vi "zadanie_4.vi"() -> ()   [LabVIEW 2020]
panel:
  in  "stop":bool
  out "S.O.S.":bool
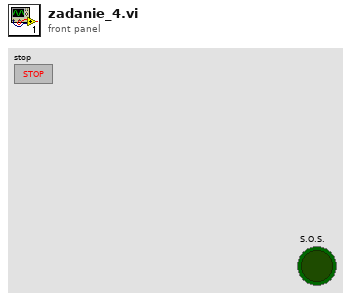
[diagram p1: front panel]
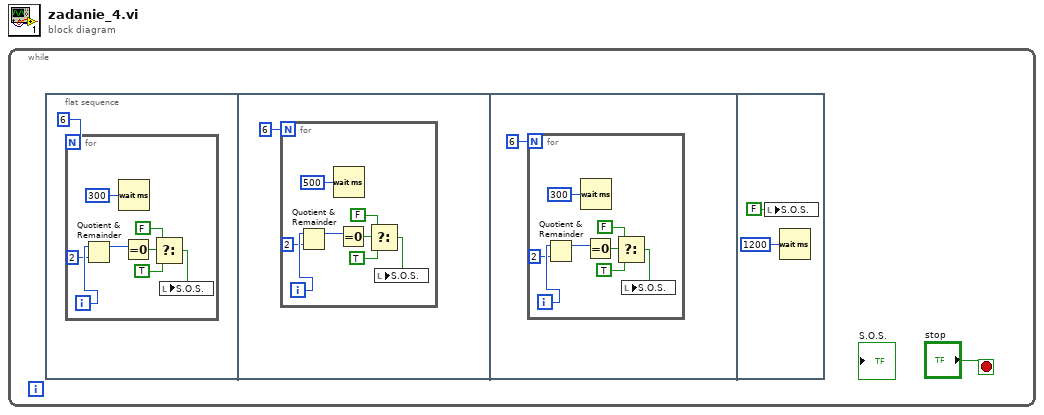
[diagram p0: block diagram]
diagram:
  n1 = while {
    stop <- "stop" stop-if-true
    n2 = flat-sequence {
      frame #0 {
        n3 = for {
          N: 6 -> [_]
          i -> [w9]
          n4 = Quotient & Remainder(x=w9, y=2) -> (x-y*floor(x/y)=w7:i32)  [unwired: 1 out]
          n5 = Wait (ms)(milliseconds to wait=u32 300) -> ()  [unwired: 1 out]
          n6 = Equal To 0?(x=w7) -> (x = 0?=w6:bool)
          n7 = Select(t=FALSE, s=w6, f=TRUE) -> (s? t:f=w5:bool)
          n8 = local write "S.O.S."(w5) -> ()
        }
      }
      frame #1 {
        n9 = for {
          N: 6 -> [_]
          i -> [w18]
          n10 = Quotient & Remainder(x=w18, y=2) -> (x-y*floor(x/y)=w16:i32)  [unwired: 1 out]
          n11 = Wait (ms)(milliseconds to wait=u32 500) -> ()  [unwired: 1 out]
          n12 = Equal To 0?(x=w16) -> (x = 0?=w15:bool)
          n13 = Select(t=FALSE, s=w15, f=TRUE) -> (s? t:f=w14:bool)
          n14 = local write "S.O.S."(w14) -> ()
        }
      }
      frame #2 {
        n15 = for {
          N: 6 -> [_]
          i -> [w27]
          n16 = Quotient & Remainder(x=w27, y=2) -> (x-y*floor(x/y)=w25:i32)  [unwired: 1 out]
          n17 = Wait (ms)(milliseconds to wait=u32 300) -> ()  [unwired: 1 out]
          n18 = Equal To 0?(x=w25) -> (x = 0?=w24:bool)
          n19 = Select(t=FALSE, s=w24, f=TRUE) -> (s? t:f=w23:bool)
          n20 = local write "S.O.S."(w23) -> ()
        }
      }
      frame #3 {
        n21 = local write "S.O.S."(FALSE ("S.O.S.")) -> ()
        n22 = Wait (ms)(milliseconds to wait=u32 1200) -> ()  [unwired: 1 out]
      }
    }
  }
